vi "S2C_XML_UpdateMeasStatus.vi"(8 "Error In":errorcluster, 11 "Result":string) -> (0 "Error Out":errorcluster)   [LabVIEW 2015]
uses:
  S2C_XML_Globals.vi
  <vilib>/xml/Close Reference(Node).vi
  <resource>/objmgr/DOMUserDefRef.rc
  <vilib>/xml/NI_XML.lvlib
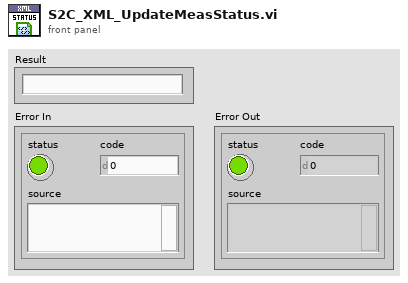
[diagram p1: front panel]
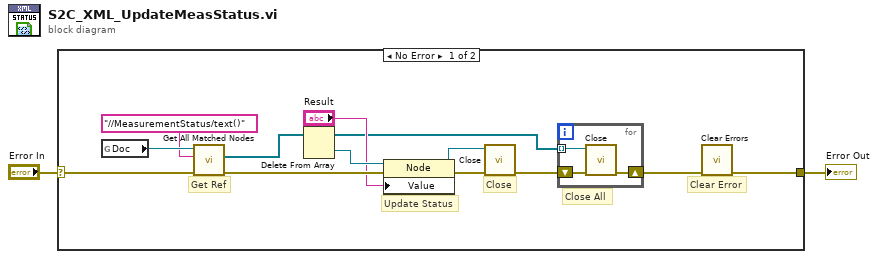
[diagram p0: block diagram]
diagram:
  n1 = case shown="No Error" "Error In" {
    selector: "Error In" -> [w13 w19]
    tunnel: [w3 w19] -> w2
    frame No Error {
      # "Clear Error"
      # "Close All"
      # "Update Status"
      # "Close"
      # "Get Ref"
      n2 = global read "S2C_XML_Globals.vi" "Doc"() -> (w15:refnum<k20>)
      n3 = call <vilib>:"Get All Matched Nodes.vi"("error in (no error)"=w13, "XPath expression"="//MeasurementStatus/text()", "node in"=w15) -> ("error out"=w14:errorcluster, "node result array"=w11:refnum<k20>[])  [unwired: 6 in, 1 out]
      n4 = Delete From Array(array=w11) -> (deleted portion=w10:refnum<k20>, array with subset deleted=w5:refnum<k20>[])  [unwired: 2 in]
      n5 = property class="Node"(reference=w10, error in=w14, "Value"="Result") -> (reference out=w8:refnum<k20>, error out=w9:errorcluster)
      n6 = call-poly <vilib>:"Close.vi"("error in (no error)"=w9, "node"=w8) -> ("error out"=w6:errorcluster)  [unwired: 7 in]
      n7 = for {
        shift-right: [w17] -> w4
        shift-left: w6 -> [w18]
        tunnel: w5 -> [w16] mode=indexing
        n8 = call-poly <vilib>:"Close.vi"("error in (no error)"=w18, "node"=w16) -> ("error out"=w17:errorcluster)  [unwired: 7 in]
      }
      n9 = call <vilib>:"Clear Errors.vi"("error in (no error)"=w4) -> ("error out"=w3:errorcluster)  [unwired: 5 in, 1 out]
    }
    frame Error {
    }
  }
  "Error Out" <- w2
